vi "Get Failure Action References.vi"(8 "error in (no error)":errorcluster, 11 "Assert Name":string) -> (0 "error out":errorcluster, 2 "Created New?":bool, 3 "Failure Action Events":T1)   [LabVIEW 2016, in "AssertEngine.lvlib"]
doc: "Creates or recovers the event and single element queue references to change the failure action."
uses:
  AssertEngine.lvlib
  Failure Action References.ctl
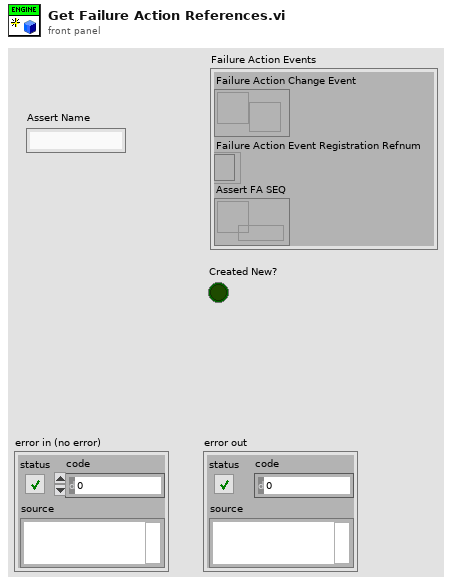
[diagram p1: front panel]
types:
  T1 = typedef "AssertEngine.lvlib/Failure Action References.ctl" = cluster{"Failure Action Change Event":refnum<user-event>, "Failure Action Event Registration Refnum":refnum<event-registration>, "Assert FA SEQ":refnum<queue>}
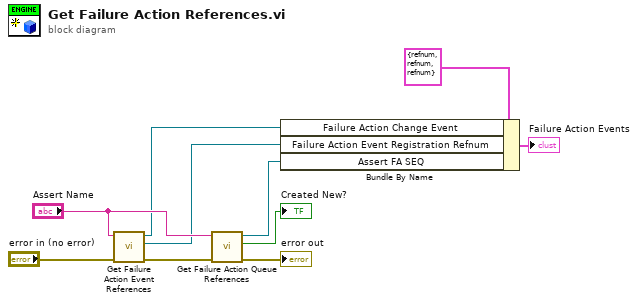
[diagram p0: block diagram]
diagram:
  n1 = call "Get Failure Action Event References.vi"("error in (no error)"="error in (no error)", "Assert Name"="Assert Name") -> ("error out"=w8:errorcluster, "Event Registration Refnum"=w4:refnum<event-registration>, "Failure Action Change Event"=w5:refnum<user-event>)  [unwired: 7 in]
  n2 = call "Get Failure Action Queue References.vi"("error in (no error)"=w8, "Assert Name"="Assert Name") -> ("error out"=→"error out":errorcluster, "created new?"=→"Created New?":bool, "Assert FA SEQ"=w3:refnum<queue>)  [unwired: 7 in]
  n3 = Bundle By Name(cluster=T1 {"Failure Action Change Event"=refnum, "Failure Action Event Registration Refnum"=refnum, "Assert FA SEQ"=refnum}, "Failure Action Change Event"=w5, "Failure Action Event Registration Refnum"=w4, "Assert FA SEQ"=w3) -> (→"Failure Action Events":T1)
